vi "Determine if Executable.vi"(1 "Path":path) -> (0 "EXE?":bool)   [LabVIEW 2012]
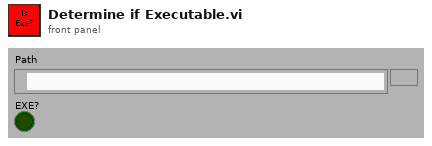
[diagram p1: front panel]
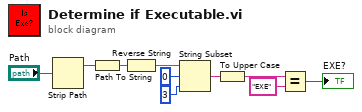
[diagram p0: block diagram]
diagram:
  n1 = Strip Path(path="Path") -> (stripped path=w9:path)  [unwired: 1 out]
  n2 = Path To String(path=w9) -> (string=w8:string)
  n3 = Reverse String(1:w8) -> (0:w7:string)
  n4 = String Subset(string=w7, offset (0)=0, length (rest)=3 ("length (rest)")) -> (substring=w4:string)
  n5 = To Upper Case(1:w4) -> (0:w3:string)
  n6 = Equal?(x=w3, y="EXE") -> (x = y?=→"EXE?":bool)
